vi "Update MSG.vi"(8 "error in (no error)":errorcluster, 10 "MSG":string, 11 "MSG in":refnum<class "MSG.lvclass">) -> (0 "error out":errorcluster, 3 "MSG out":refnum<class "MSG.lvclass">)   [LabVIEW 2020, in "MSG.lvlib" / "MSG.lvclass"]
uses:
  MSG.lvclass
  MSG.lvclass/MSG.ctl
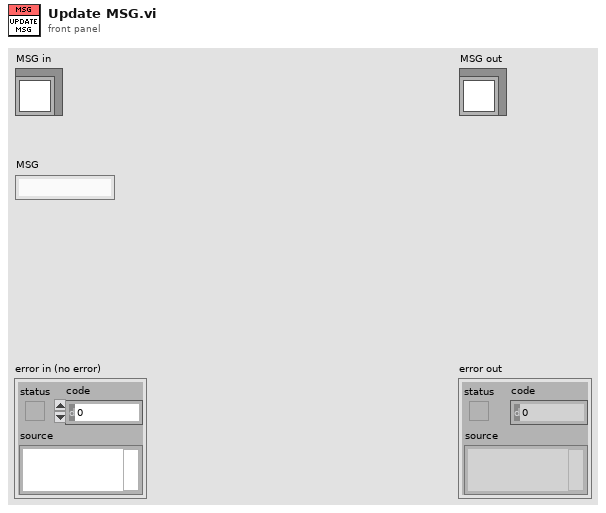
[diagram p1: front panel]
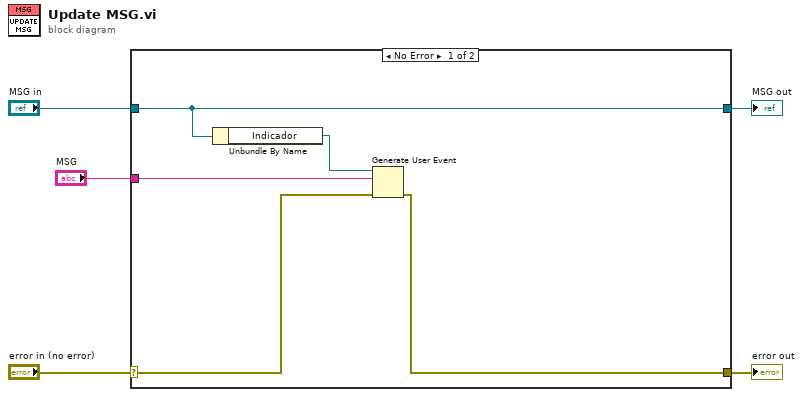
[diagram p0: block diagram]
diagram:
  n1 = case shown="No Error" "error in (no error)" {
    selector: "error in (no error)" -> [w7 w12]
    tunnel: [w6 w12] -> w4
    tunnel: [w10 w11] -> w2
    tunnel: "MSG in" -> [w10 w11]
    tunnel: "MSG" -> [w9 _]
    frame No Error {
      n2 = Unbundle By Name(w10) -> ("Indicador"=w8:refnum<user-event>)
      n3 = Generate User Event(user event=w8, event data cluster=w9, error in=w7) -> (error out=w6:errorcluster)  [unwired: 1 in, 1 out]
    }
    frame Error {
    }
  }
  "error out" <- w4
  "MSG out" <- w2
